vi "Configure Record Data (Manual).vi"(0 "VISA resource name":refnum<visa-resource-name>, 5 "Record Number (1)":i32=1 min=1 max=440 step=1, 7 "Kind of Channel (0: Off)":u16(ring) items=["Off", "IO", "Math", "Com"], 9 "Channel Number (0001)":string="0001", 11 "error in (no error)":errorcluster) -> (4 "VISA resource name out":refnum<visa-resource-name>, 6 "Record Number":i32, 15 "error out":errorcluster)   [LabVIEW 2020, in "Yokogawa GX Series.lvlib"]
doc: "Sets the channel for recording manual sampled data.\n\nCommand: SRecManual"
uses:
  <instrlib>/Yokogawa GX Series/Yokogawa GX Series.lvlib
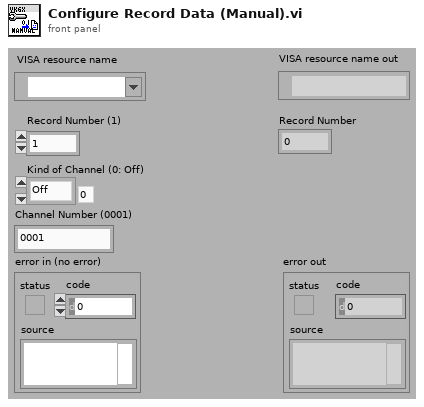
[diagram p1: front panel]
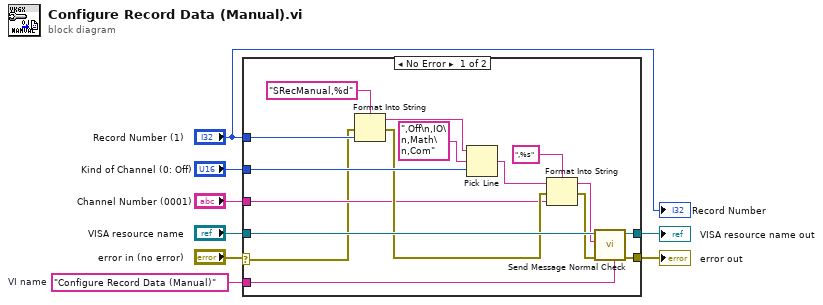
[diagram p0: block diagram]
diagram:
  w8 = "Configure Record Data (Manual)"  # VI name
  n1 = case shown="No Error" "error in (no error)" {
    selector: "error in (no error)" -> [w9 w25]
    tunnel: w8 -> [w23 _]
    tunnel: "VISA resource name" -> [w22 w26]
    tunnel: [w21 w26] -> w6
    tunnel: [w20 w25] -> w5
    tunnel: "Kind of Channel (0: Off)" -> [w18 _]
    tunnel: "Record Number (1)" -> [w17 _]
    tunnel: "Channel Number (0001)" -> [w12 _]
    frame No Error {
      n2 = Format Into String(format string="SRecManual,%d", error in=w9, w17) -> (resulting string=w19:string, error out=w13:errorcluster)  [unwired: 1 in]
      n3 = Pick Line(string ("")=w19, multi-line string=",Off\n,IO\n,Math\n,Com", line index=w18) -> (output string=w15:string)
      n4 = Format Into String(format string=",%s", initial string=w15, error in=w13, w12) -> (resulting string=w10:string, error out=w11:errorcluster)
      n5 = call <instrlib>:"Send Message Normal Check.vi"("Source (\"\")"=w23, "error in (no error)"=w11, "Send Message (\"\")"=w10, "VISA resource name"=w22) -> ("error out"=w20:errorcluster, "VISA resource name out"=w21:refnum<visa-resource-name>)  [unwired: 1 in, 5 out]
    }
    frame Error {
    }
  }
  "error out" <- w5
  "VISA resource name out" <- w6
  "Record Number" <- "Record Number (1)"
